vi "MerweScSigPts_New.vi"(8 "Kappa":i32, 9 "Beta":dbl, 10 "Alpha":dbl, 11 "States":i32) -> (3 "MerweScaledSigmaPts":T1)   [LabVIEW 2019, in "Trajectory_Library.lvlib"]
doc: "Generates sigma points and weights according to Van der Merwe's 2004 dissertation[1] for the UnscentedKalmanFilter class.\n \nIt parametrizes the sigma points using alpha, beta, kappa terms, and is the version seen in most publications. Unless you know better, this should be your default choice.\n \nStates is the dimensionality of the state. 2*States+1 weights will be generated.\n \n[1] R. Van der Merwe \"Sigma-Point Kalman Filters for Probabilitic Inference in Dynamic State-Space Models\" (Doctoral dissertation)\n\nConstructs a generator for Van der Merwe scaled sigma points.\n \nInputs:\n - states -- the number of states.\n - alpha -- Determines the spread of the sigma points around the mean. Usually a small\n positive value (1e-3).\n - beta -- Incorporates prior knowledge of the distribution of the mean. For Gaussian\n distributions, beta = 2 is optimal.\n - kappa -- Secondary scaling parameter usually set to 0 or 3 - States.\n\nOutputs:\n - MerweScaledSigmaPts -- data cluster"
uses:
  Trajectory_Library.lvlib
  TypeDef/MERWE_SCALED_SIGMA_PTS.ctl
  <vilib>/Analysis/Matrix/Datatypes/RealMatrix.ctl
  <vilib>/Analysis/Matrix/NI_Matrix.lvlib
panel:
  # "<?, 1>"
  # "<?, 1>"
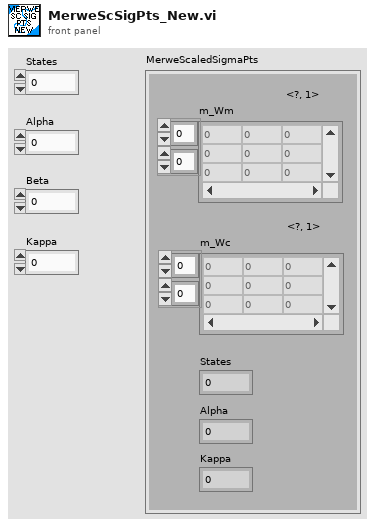
[diagram p1: front panel]
types:
  T1 = typedef "Trajectory_Library.lvlib/MERWE_SCALED_SIGMA_PTS.ctl" = cluster{"m_Wm":T2, "States":i32, "Alpha":dbl, "m_Wc":T2, "Kappa":i32}
  T2 = typedef "NI_Matrix.lvlib/RealMatrix.ctl" = dbl[][]
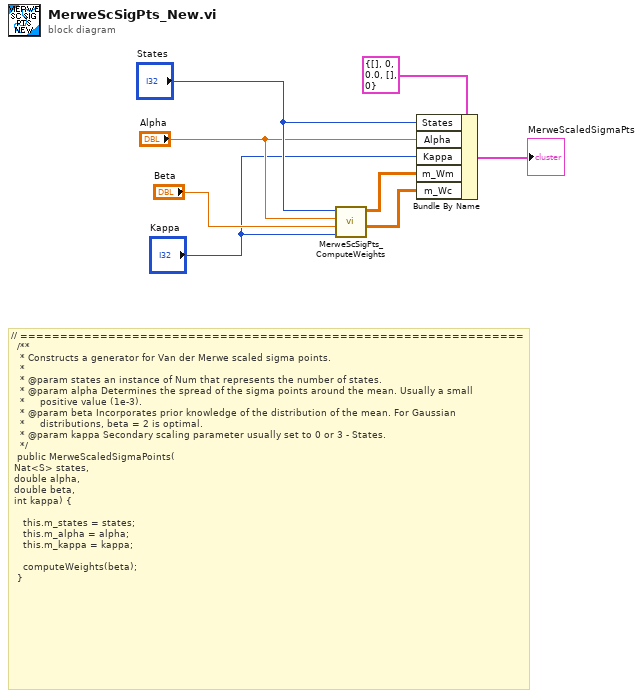
[diagram p0: block diagram]
diagram:
  # "// ===============================================================\n  /**\n   * Constructs a generator for Van der Merwe scaled sigma points.\n   *\n   * @param states an instance of Num that represents the number of states.\n   * @param alpha Determines the spread of the sigma points around the mean. Usually a small\n   *     positive value (1e-3).\n   * @param beta Incorporates prior knowledge of the distribution of the mean. For Gaussian\n   *     distributions, beta = 2 is optimal.\n   * @param kappa Secondary scaling parameter usually set to 0 or 3 - States.\n   */\n  public MerweScaledSigmaPoints(\n\tNat<S> states, \n\tdouble alpha, \n\tdouble beta, \n\tint kappa) {\n\n    this.m_states = states;\n    this.m_alpha = alpha;\n    this.m_kappa = kappa;\n\n    computeWeights(beta);\n  }"
  n1 = call "MerweScSigPts_ComputeWeights.vi"("Kappa"="Kappa", "Beta"="Beta", "Alpha"="Alpha", "States"="States") -> ("Wc"=w1:T2, "Wm"=w2:T2)  [unwired: 6 in]
  n2 = Bundle By Name(cluster=T1 {"m_Wm"=[], "States"=0, "Alpha"=0.0, "m_Wc"=[], "Kappa"=0} ("MERWE_SCALED_SIGMA_PTS"), "States"="States", "Alpha"="Alpha", "Kappa"="Kappa", "m_Wm"=w2, "m_Wc"=w1) -> (→"MerweScaledSigmaPts":T1)
